vi "A-H 2700 Cap.vi"(2 "Point #":i32, 3 "Instrument Address":refnum<visa-resource-name>) -> (0 "Stop":bool, 1 "Measurement":dbl[](array[numeric]) format="%.9f")   [LabVIEW 2019]
doc: "Reads Andeen Haegerling Automatic Capacitance bridge and returns the capacitance in pF. Does not use SRQ lines.\nScott Hannahs, F. Bitter National Magnet Lab, May 1993"
panel:
  in  "Return Dissapation":u8(slide) max=5 step=1 scale=0.0..5.0
  in  "AVE TIME":u32(slide)=5 max=15 step=1 scale=0.0..15.0
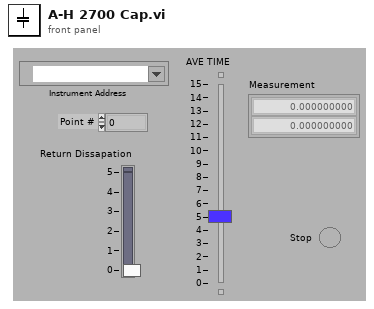
[diagram p1: front panel]
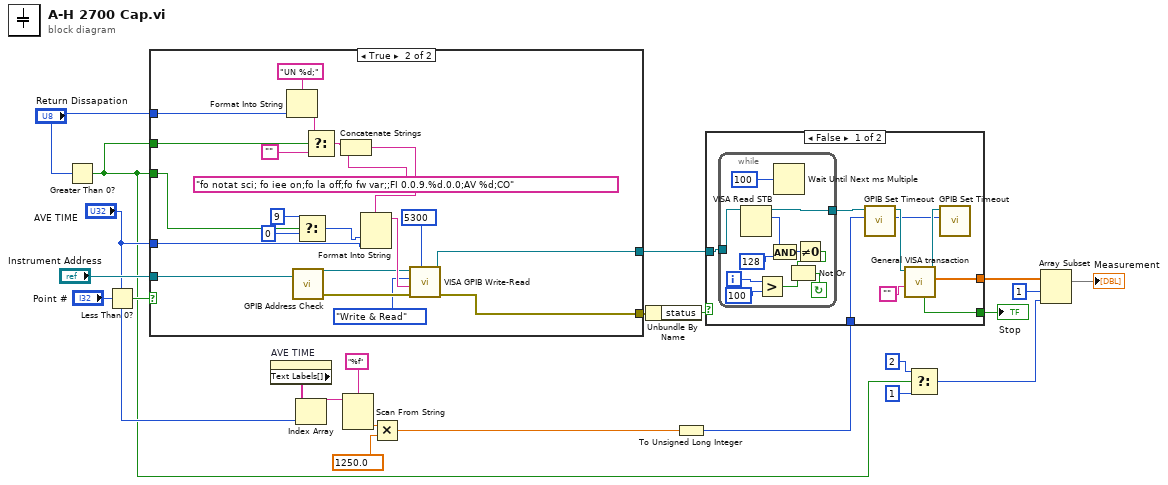
[diagram p0: block diagram]
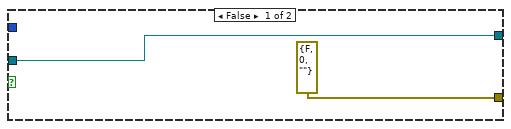
[diagram p2: hidden frame]
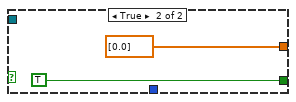
[diagram p3: hidden frame]
diagram:
  n1 = Greater Than 0?(x="Return Dissapation") -> (x > 0?=w4:bool)
  n2 = Less Than 0?(x="Point #") -> (x < 0?=w20:bool)
  n3 = case shown="True" w20 {
    tunnel: [w25 w42] -> w19
    tunnel: "Instrument Address" -> [w25 w28]
    tunnel: [errorcluster {"status"=FALSE, "code"=0, "source"=""} ("error out") w26] -> w22
    tunnel: "AVE TIME" -> [_ w33]
    tunnel: "Return Dissapation" -> [_ w36]
    tunnel: w4 -> [_ w34]
    tunnel: w4 -> [_ w29]
    frame False {
    }
    frame True {
      n4 = Format Into String(format string="UN %d;" ("Input String"), w36) -> (resulting string=w38:string)  [unwired: 2 in, 1 out]
      n5 = call "GPIB Address Check.vi"("Instrument Address"=w28) -> ("dup VISA session"=w43:refnum<visa-resource-name>, "error out"=w46:errorcluster)  [unwired: 1 in, 1 out]
      n6 = Select(t=9, s=w29, f=0) -> (s? t:f=w31:i32)
      n7 = Select(t=w38, s=w34, f="") -> (s? t:f=w40:string)
      n8 = Concatenate Strings(w40, "fo notat sci; fo iee on;fo la off;fo fw var;;FI 0.0.9.%d.0.0;AV %d;CO") -> (w35:string)
      n9 = Format Into String(format string=w35, w31, w33) -> (resulting string=w45:string)  [unwired: 2 in, 1 out]
      n10 = call "VISA GPIB Write-Read.vi"("Wait (ms)"=u32 5300 ("wait (mS)"), "error in (no error)"=w46, "Command"=w45, "Action"=enum16{"Write", "Read", "Write & Read"}."Write & Read", "VISA resource name"=w43) -> ("error out"=w26:errorcluster, "dup VISA Session"=w42:refnum<visa-resource-name>)  [unwired: 3 in, 2 out]
    }
  }
  n11 = property on="AVE TIME" class="Slide (strict)"() -> ("Text Labels[]"=w9:string[])  [unwired: 2 in, 2 out]
  n12 = Index Array(array=w9, index="AVE TIME") -> (element=w10:string)
  n13 = Scan From String(format string="%f" ("Format String"), input string=w10) -> (output 1=w12:dbl)  [unwired: 3 in, 3 out]
  n14 = Multiply(x=w12, y=1250.0) -> (x*y=w14:dbl)
  n15 = Unbundle By Name(w22) -> ("status"=w23:bool)
  n16 = To Unsigned Long Integer(number=w14) -> (unsigned 32bit integer=w7:u32)
  n17 = case shown="False" w23 {
    tunnel: w19 -> [w52 _]
    tunnel: [w55 dbl[] [0.0]] -> w17
    tunnel: [w54 TRUE ("Stop")] -> w16
    tunnel: w7 -> [w50 _]
    frame False {
      n18 = while {
        tunnel: [w57] -> w51
        tunnel: w52 -> [w56]
        i -> [w64]
        stop <- w62 continue-if-true
        n19 = VISA Read STB(11:w56) -> (2:w58:u16, 3:w57:refnum<visa-resource-name>)  [unwired: 1 in, 1 out]
        n20 = Greater?(x=w64, y=100) -> (0:w61:bool)
        n21 = And(x=w58, y=u16 128) -> (x .and. y?=w59:u16)
        n22 = Wait Until Next ms Multiple(millisecond multiple=u32 100) -> ()  [unwired: 1 out]
        n23 = Not Equal To 0?(x=w59) -> (x != 0?=w60:bool)
        n24 = Not Or(1:w61, 2:w60) -> (0:w62:bool)
      }
      n25 = call "GPIB Set Timeout.vi"("Timeout"=w50, "VISA resource name"=w51) -> ("Old Timeout"=w47:u32, "dup VISA resource name"=w49:refnum<visa-resource-name>)  [unwired: 3 in, 1 out]
      n26 = call "General VISA transaction.vi"("Command String"="", "VISA Session"=w49) -> ("Measurement"=w55:dbl[], "dup VISA Session"=w48:refnum<visa-resource-name>, "Stop"=w54:bool)  [unwired: 4 in, 3 out]
      n27 = call "GPIB Set Timeout.vi"("Timeout"=w47, "VISA resource name"=w48) -> ()  [unwired: 3 in, 3 out]
    }
    frame True {
    }
  }
  "Stop" <- w16
  n28 = Select(t=2 ("index"), s=w4, f=1 ("index")) -> (s? t:f=w3:i32)
  n29 = Array Subset(array=w17, index=1, length=w3) -> (→"Measurement":dbl[])
